vi "Rearrange DLL Output (SubVI).vi"(11 "outData":i32[](array[numeric])) -> (3 "Stimulus Parameters":dbl[][](array[numeric]))   [LabVIEW 2020]
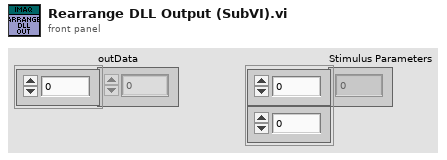
[diagram p1: front panel]
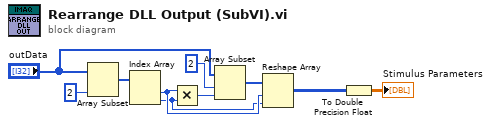
[diagram p0: block diagram]
diagram:
  n1 = Array Subset(array="outData", length=2) -> (w9:i32[])  [unwired: 1 in]
  n2 = Index Array(array=w9) -> (element #1=w2:i32, element #2=w1:i32)  [unwired: 2 in]
  n3 = Multiply(x=w2, y=w1) -> (x*y=w6:i32)
  n4 = Array Subset(array="outData", index=2, length=w6) -> (w8:i32[])
  n5 = Reshape Array(w8, w2, w1) -> (w3:i32[][])
  n6 = To Double Precision Float(number=w3) -> (double precision float=→"Stimulus Parameters":dbl[][])
